vi "Slow_movement.vi"(8 "Previous value (Shift register input)":dbl, 9 "Input":dbl, 11 "Speed (°/loop)":dbl=0.1 format="%#_13g") -> (0 "Output":dbl)   [LabVIEW 2021]
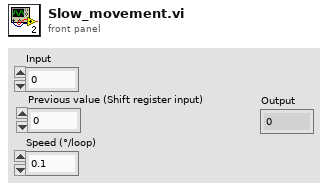
[diagram p1: front panel]
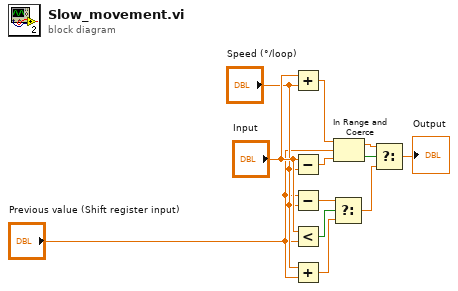
[diagram p0: block diagram]
diagram:
  n1 = Add(x="Input", y="Speed (°/loop)") -> (x+y=w5:dbl)
  n2 = Subtract(x="Input", y="Speed (°/loop)") -> (x-y=w4:dbl)
  n3 = Subtract(x="Previous value (Shift register input)", y="Speed (°/loop)") -> (x-y=w12:dbl)
  n4 = Less?(x="Input", y="Previous value (Shift register input)") -> (x < y?=w8:bool)
  n5 = Add(x="Speed (°/loop)", y="Previous value (Shift register input)") -> (x+y=w11:dbl)
  n6 = Select(t=w12, s=w8, f=w11) -> (s? t:f=w9:dbl)
  n7 = In Range and Coerce(upper limit=w5, x="Previous value (Shift register input)", lower limit=w4) -> (coerced(x)=w7:dbl, In Range?=w10:bool)
  n8 = Select(t=w7, s=w10, f=w9) -> (s? t:f=→"Output":dbl)
